vi "ArdnoManualValves.vi"() -> ()   [LabVIEW 2018, in "Arduino.lvlib"]
uses:
  Arduino.lvlib
  <vilib>/MakerHub/LINX/Public/Peripherals/Digital/Digital Write N Chans.vi
  <vilib>/MakerHub/LINX/Private/Local IO/LinxDigitalWrite.vi
  <vilib>/MakerHub/LINX/Public/Utilities/Check Channel.vi
  <vilib>/MakerHub/LINX/Public/Utilities/Open Serial.vi
  <vilib>/MakerHub/LINX/Private/Utilties/Generate Error.vi
  <vilib>/MakerHub/LINX/LMH-LINX.lvlib
panel:
  in  "Valves (A1-C7) comma seperated":string
  out "Error Out":errorcluster
  out "Device Name":string
  in  "error in (no error)":errorcluster
  in  "VISA resource name":refnum<visa-resource-name>
  out "Open?":bool
  in  "Manual Open":bool
  in  "stop":bool
  # "ALWAYS TERMINATE THE\nPROGRAM WITH THIS STOP BUTTON!"
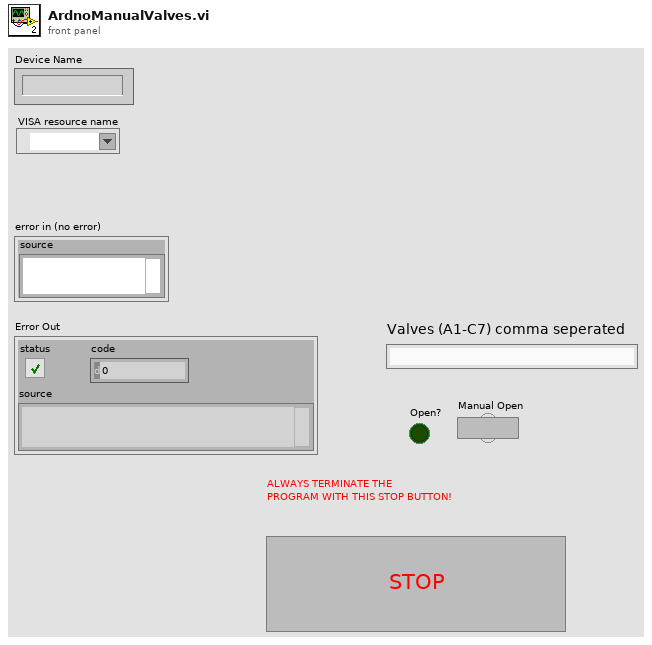
[diagram p1: front panel]
types:
  T1 = typedef "LMH-LINX.lvlib/LINX Ref.ctl" = cluster{"IO":T2, "Interface":T3, "LINX Device Config":T4}
  T2 = typedef "LMH-LINX.lvlib/Platform.ctl" = enum16{"Remote", "Local"}
  T3 = typedef "LMH-LINX.lvlib/Interface.ctl" = enum16{"Serial", "TCP"}
  T4 = typedef "LMH-LINX.lvlib/Device.lvlib/LINX Device Config.ctl" = cluster{"Interface":T3, "COM Port":refnum<visa-resource-name>, "TCP Configuration":T5, "Device Family":u8, "Device ID":u8, "Device Name":string, "TCP Ref":refnum<k5>, "Channels":T6}
  T5 = typedef "LMH-LINX.lvlib/Device.lvlib/TCP Config.ctl" = cluster{"IP Address":string, "Port":u16}
  T6 = typedef "LMH-LINX.lvlib/Channels.ctl" = cluster{"DI":u8[], "DO":u8[], "AI":u8[], "AO":u8[], "PWM":u8[], "QE":u8[], "UART":u8[], "I2C 2":u8[], "SPI":u8[], "CAN":u8[], "Servo":u8[], "AI Ref (V)":dbl, "AI Resolution (Bits)":u8, "AO Ref (V)":dbl, "AO Resolution (Bits)":u8}
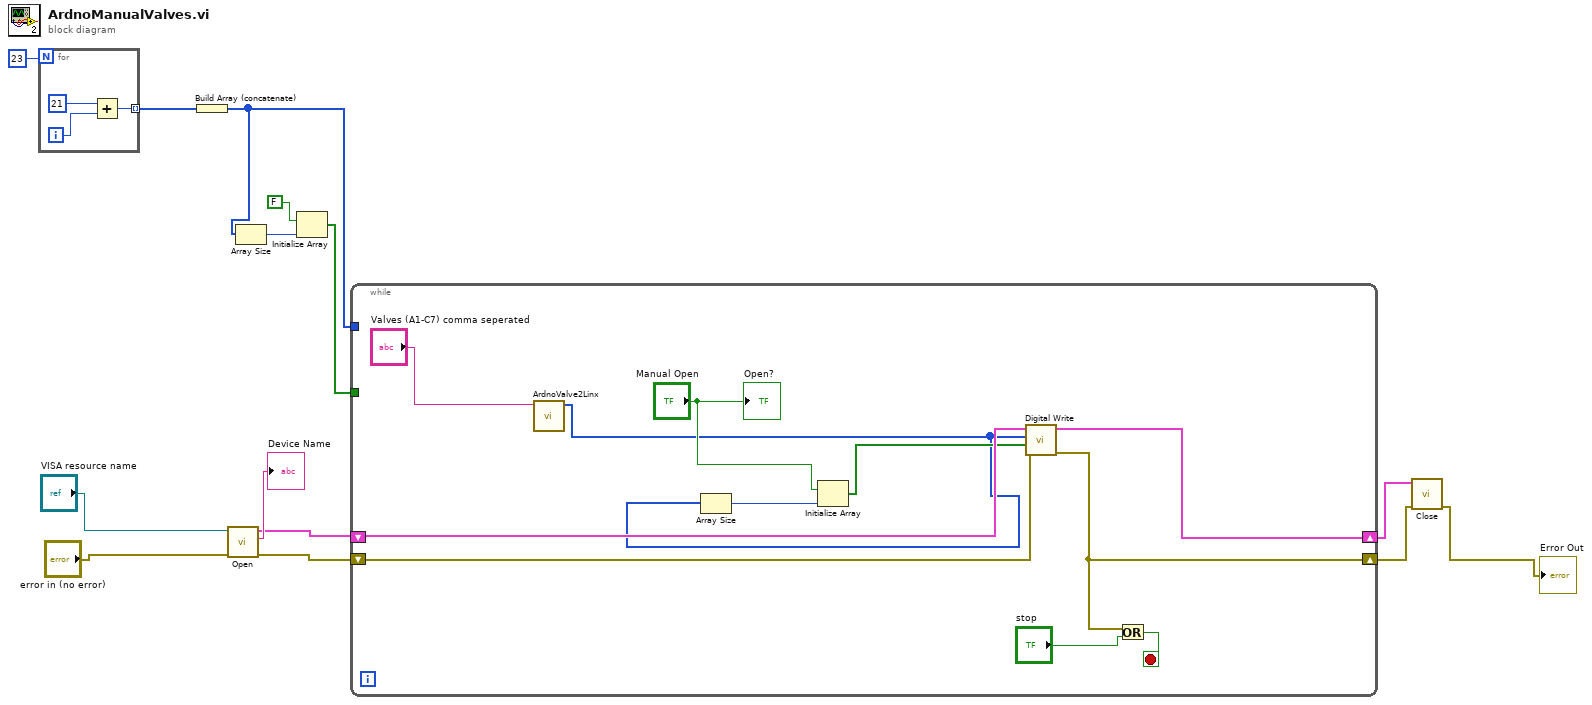
[diagram p0: block diagram]
diagram:
  n1 = for {
    N: 23 -> [_]
    tunnel: [w15] -> w13 mode=indexing
    i -> [w17]
    n2 = Add(x=21, y=w17) -> (x+y=w15:i32)
  }
  n3 = Build Array (concatenate)(w13) -> (w12:i32[])
  n4 = call-poly <vilib>:"Open.vi"("Error In"="error in (no error)", "Serial Port"="VISA resource name") -> ("Error Out"=w3:errorcluster, "Device Name"=→"Device Name":string, "LINX Resource"=w1:T1)  [unwired: 7 in]
  n5 = Array Size(array=w12) -> (size(s)=w11:i32)
  n6 = Initialize Array(FALSE, w11) -> (w9:bool[])
  n7 = while {
    tunnel: w12 -> [_]
    tunnel: w9 -> [_]
    shift-right: [w20] -> w8
    shift-left: w1 -> [w24]
    shift-right: [w21] -> w7
    shift-left: w3 -> [w22]
    stop <- w27 stop-if-true
    n8 = call "ArdnoValve2Linx.vi"("Valve (A1-C8),\n comma separated"="Valves (A1-C7) comma seperated") -> ("Linx Port"=w18:i32[])  [unwired: 8 in, 2 out]
    n9 = Array Size(array=w18) -> (size(s)=w26:i32)
    n10 = Initialize Array("Manual Open", w26) -> (w23:bool[])
    n11 = call-poly <vilib>:"Digital Write.vi"("Error In"=w22, "Values"=w23, "DO Channels"=w18, "LINX Resource"=w24) -> ("Error Out"=w21:errorcluster, "LINX Resource"=w20:T1)  [unwired: 6 in]
    n12 = Or(x=w21, y="stop") -> (x .or. y?=w27:bool)
    "Open?" <- "Manual Open"
  }
  n13 = call <vilib>:"Close.vi"("Error In"=w7, "LINX Resource"=w8) -> ("Error Out"=→"Error Out":errorcluster)  [unwired: 9 in]
